vi "ArmTest_RLE_and_XYZ.vi"() -> ()   [LabVIEW 2020]
uses:
  <vilib>/Rock Robotics/WPI/ThirdParty/JAS_Junk/TrajLib/Trajectory_Library.lvlib
panel:
  out "Passed":bool
  out "Extend 2":dbl
  out "Lift 2":dbl
  out "Rotate 2":dbl
  out "z":dbl
  out "y":dbl
  out "x":dbl
  in  "Rotate":dbl
  in  "Lift":dbl
  in  "Extend":dbl
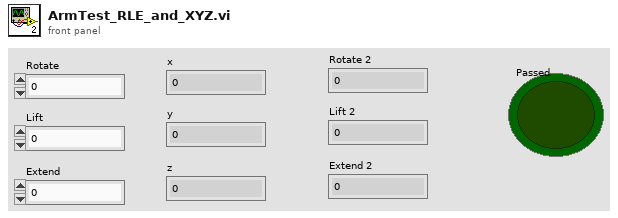
[diagram p1: front panel]
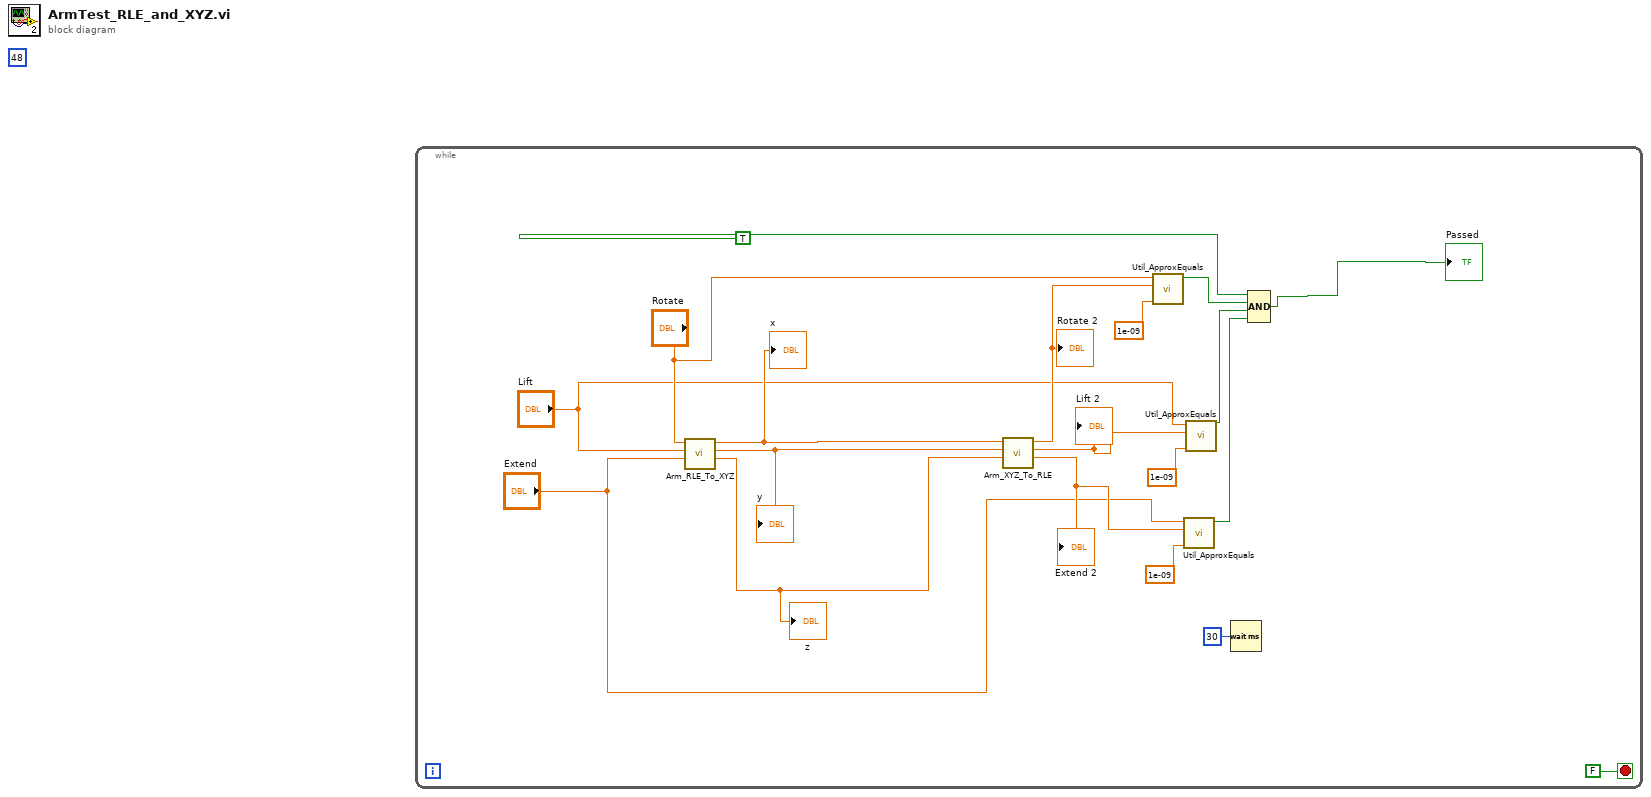
[diagram p0: block diagram]
diagram:
  (unwired) 48
  n1 = while {
    stop <- FALSE stop-if-true
    n2 = call "Arm_RLE_To_XYZ.vi"("Extend"="Extend", "Lift"="Lift", "Rotate"="Rotate") -> ("z"=w15:dbl, "y"=w16:dbl, "x"=w17:dbl)  [unwired: 6 in]
    "x" <- w17
    "y" <- w16
    "z" <- w15
    n3 = call "Arm_XYZ_To_RLE.vi"("Z"=w15, "Y"=w16, "X"=w17) -> ("Extend"=w9:dbl, "Lift"=w10:dbl, "Rotate"=w11:dbl)  [unwired: 6 in]
    "Rotate 2" <- w11
    "Lift 2" <- w10
    "Extend 2" <- w9
    n4 = call <vilib>:"Util_ApproxEquals.vi"("Tolerance"=1e-09, "Value 2"=w11, "Value 1"="Rotate") -> ("ApproxEquals"=w8:bool)  [unwired: 8 in]
    n5 = call <vilib>:"Util_ApproxEquals.vi"("Tolerance"=1e-09, "Value 2"=w9, "Value 1"="Extend") -> ("ApproxEquals"=w6:bool)  [unwired: 8 in]
    n6 = call <vilib>:"Util_ApproxEquals.vi"("Tolerance"=1e-09, "Value 2"=w10, "Value 1"="Lift") -> ("ApproxEquals"=w7:bool)  [unwired: 8 in]
    n7 = Wait (ms)(milliseconds to wait=u32 30) -> ()  [unwired: 1 out]
    n8 = Compound Arithmetic op=AND(TRUE, w8, w7, w6) -> (→"Passed":bool)
  }
